vi "waitTarget-X.vi"(0 "Device in X":refnum<k24>, 5 "GetPOS X":refnum<vi>, 7 "Position X":sgl, 9 "GetPOS Y":refnum<vi>, 11 "Device in Y":refnum<k24>, 12 "Position Y":sgl) -> (4 "Device out X":refnum<k24>, 6 "GetPOS X":dbl format="%#_6f", 8 "GetPOS Y":dbl format="%#_6f", 15 "Device out Y":refnum<k24>)   [LabVIEW 2014]
doc: "André Romero - 2018\nandretec@ifsc.usp.br"
uses:
  C:/user-Lab/AndreTec/GITs/andretec/Thorlabs-Vector-Move/kinesisTec/Kinesis/Thorlabs.MotionControl.TCube.DCServoCLI.dll
  kinesisTec/Kinesis/Thorlabs.MotionControl.TCube.DCServoCLI.dll
panel:
  in  "error":dbl=0.004 format="%#_13g"
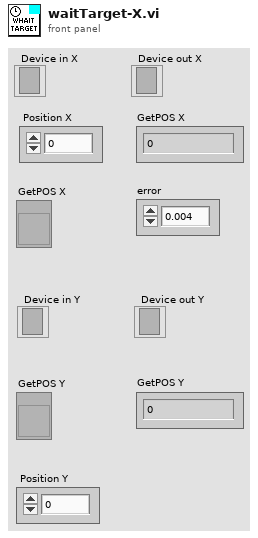
[diagram p1: front panel]
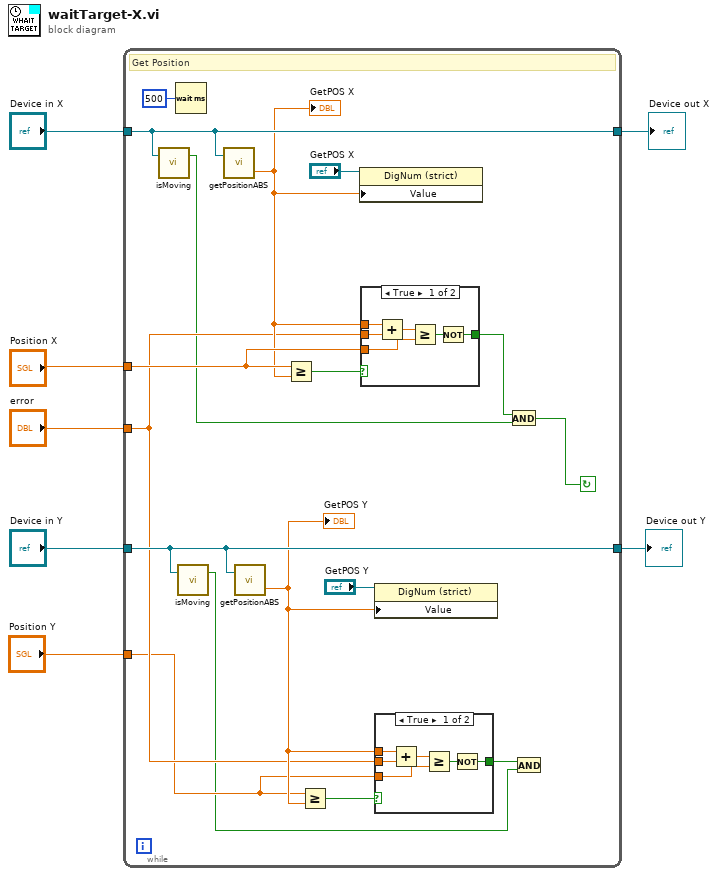
[diagram p0: block diagram]
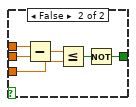
[diagram p2: hidden frame]
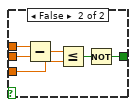
[diagram p3: hidden frame]
diagram:
  n1 = while {
    tunnel: "Device in X" -> [w24]
    tunnel: [w24] -> w6
    tunnel: "Position X" -> [w20]
    tunnel: "error" -> [w14]
    tunnel: "Device in Y" -> [w17]
    tunnel: [w17] -> w2
    tunnel: "Position Y" -> [w13]
    stop <- w8 continue-if-true
    # "Get Position"
    n2 = call "isMoving.vi"("Device in"=w24) -> ("IsMoving"=w9:bool)  [unwired: 1 in, 1 out]
    n3 = Wait (ms)(milliseconds to wait=u32 500) -> ()  [unwired: 1 out]
    n4 = call "isMoving.vi"("Device in"=w17) -> ("IsMoving"=w12:bool)  [unwired: 1 in, 1 out]
    n5 = call "getPositionABS.vi"("Device"=w24) -> ("GetPOS"=w19:dbl)  [unwired: 1 in, 1 out]
    "GetPOS X" <- w19
    n6 = call "getPositionABS.vi"("Device"=w17) -> ("GetPOS"=w15:dbl)  [unwired: 1 in, 1 out]
    "GetPOS Y" <- w15
    n7 = Greater Or Equal?(x=w20, y=w19) -> (x >= y?=w21:bool)
    n8 = Greater Or Equal?(x=w13, y=w15) -> (x >= y?=w16:bool)
    n9 = property class="DigNum (strict)"(reference="GetPOS X", "Value"=w19) -> ()  [unwired: 1 in, 2 out]
    n10 = case shown="True" w21 {
      tunnel: w19 -> [w42 w48]
      tunnel: w14 -> [w41 w47]
      tunnel: w20 -> [w39 w45]
      tunnel: [w37 w43] -> w10
      frame True {
        n11 = Add(x=w42, y=w41) -> (x+y=w40:dbl)
        n12 = Greater Or Equal?(x=w40, y=w39) -> (x >= y?=w38:bool)
        n13 = Not(x=w38) -> (.not. x?=w37:bool)
      }
      frame False {
        n14 = Subtract(x=w48, y=w47) -> (x-y=w46:dbl)
        n15 = Less Or Equal?(x=w46, y=w45) -> (x <= y?=w44:bool)
        n16 = Not(x=w44) -> (.not. x?=w43:bool)
      }
    }
    n17 = property class="DigNum (strict)"(reference="GetPOS Y", "Value"=w15) -> ()  [unwired: 1 in, 2 out]
    n18 = case shown="True" w16 {
      tunnel: w15 -> [w30 w36]
      tunnel: w14 -> [w29 w35]
      tunnel: w13 -> [w27 w33]
      tunnel: [w25 w31] -> w11
      frame True {
        n19 = Add(x=w30, y=w29) -> (x+y=w28:dbl)
        n20 = Greater Or Equal?(x=w28, y=w27) -> (x >= y?=w26:bool)
        n21 = Not(x=w26) -> (.not. x?=w25:bool)
      }
      frame False {
        n22 = Subtract(x=w36, y=w35) -> (x-y=w34:dbl)
        n23 = Less Or Equal?(x=w34, y=w33) -> (x <= y?=w32:bool)
        n24 = Not(x=w32) -> (.not. x?=w31:bool)
      }
    }
    n25 = And(x=w10, y=w9) -> (x .and. y?=w8:bool)
    n26 = And(x=w11, y=w12) -> ()  [unwired: 1 out]
  }
  "Device out X" <- w6
  "Device out Y" <- w2
